vi "SelectElementToWrite.vi"(8 "error in (no error)":errorcluster, 11 "BaseAccessorScripter in":refnum<class "BaseAccessorScripter.lvclass">) -> (0 "error out":errorcluster, 3 "BaseAccessorScripter out":refnum<class "BaseAccessorScripter.lvclass">)   [LabVIEW 2021, in "MemberVICreation.lvlib" / "BaseAccessorScripter.lvclass"]
uses:
  <resource>/Framework/Providers/LVClassLibrary/NewAccessors/BaseAccessorScripter/BaseAccessorScripter.lvclass
  <resource>/Framework/Providers/LVClassLibrary/NewAccessors/BaseAccessorScripter/BaseAccessorScripter.lvclass/BaseAccessorScripter.ctl
  <resource>/Framework/Providers/LVClassLibrary/NewAccessors/MemberVICreation.lvlib
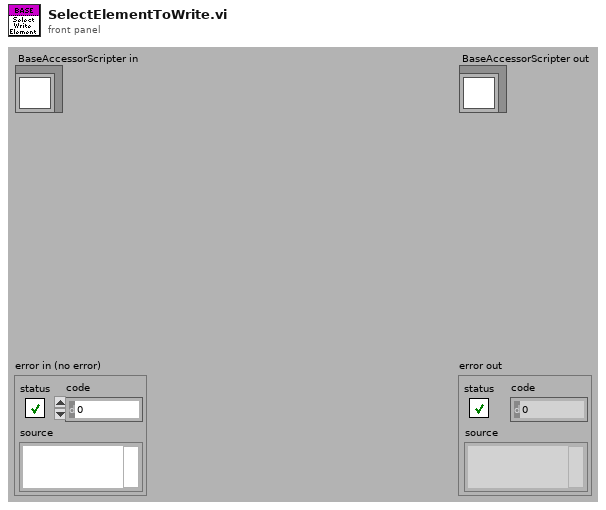
[diagram p1: front panel]
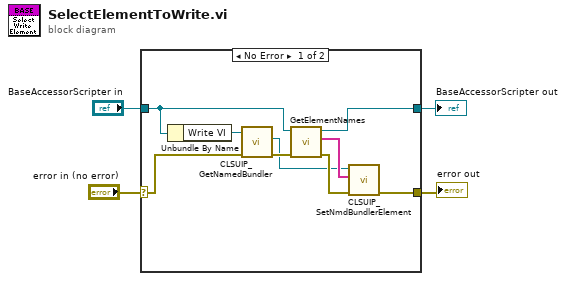
[diagram p0: block diagram]
diagram:
  n1 = case shown="No Error" "error in (no error)" {
    selector: "error in (no error)" -> [w12 w15]
    tunnel: [w5 w15] -> w3
    tunnel: [w10 w14] -> w1
    tunnel: "BaseAccessorScripter in" -> [w11 w14]
    frame No Error {
      n2 = Unbundle By Name(w11) -> ("Write VI"=w13:refnum<vi>)
      n3 = call <resource>:"CLSUIP_GetNamedBundler.vi"("error in (no error)"=w12, "VI Refnum"=w13) -> ("error out"=w9:errorcluster, "NmdBundler Ref"=w6:refnum<vi>)  [unwired: 8 out]
      n4 = call-dynamic "GetElementNames.vi"("error in (no error)"=w9, "BaseAccessorScripter in"=w11) -> ("error out"=w8:errorcluster, "Element Names"=w7:string[], "BaseAccessorScripter out"=w10:refnum<class "BaseAccessorScripter.lvclass">)  [unwired: 7 out]
      n5 = call <resource>:"CLSUIP_SetNmdBundlerElement.vi"("error in (no error)"=w8, "Element Names"=w7, "NmdBundler Ref"=w6) -> ("error out"=w5:errorcluster)  [unwired: 8 out]
    }
    frame Error {
    }
  }
  "error out" <- w3
  "BaseAccessorScripter out" <- w1
